vi "can test.vi"() -> ()   [LabVIEW 2015]
uses:
  <vilib>/FPGAPlugInAG/cRIO-9030/niLvFpga_Open_cRIO-9030.vi
  <vilib>/rvi/interface/common/dynamic/niFpgaDynamicAddResources.vi
  <vilib>/FPGAPlugInAG/Dynamic/niLvFpga_Abort_Dynamic.vi
  <vilib>/FPGAPlugInAG/Dynamic/niLvFpga_Run_Dynamic.vi
  <vilib>/Utility/error.llb/Error Cluster From Error Code.vi
  <vilib>/rvi/errors/niLvFpgaAdjustHostInterfaceError.vi
  <vilib>/rvi/interface/nirviOpenFPGA/nirviOpenFPGA.xnode
  FPGA Bitfiles/autonomous_FPGATarget4_fpga1_rudp+OsNkSQ.lvbitx
  samsung/fpga 1.vi
  <vilib>/rvi/interface/nirviMethod/nirviMethod.xnode
  <vilib>/FPGAPlugInAG/Dynamic/niLvFpga_ReadFifo_Dynamic.vi
  <vilib>/rvi/errors/niLvFpgaMergeErrorWithErrorCode.vi
  <vilib>/NI_Real-Time Target Support.lvlib
panel:
  out "tic":u32
  out "filesave":refnum<file>
  out "CAN_time 10":u32
  out "FPGA":refnum<k20>
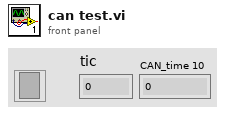
[diagram p1: front panel]
types:
  T1 = enum16{"open", "replace", "create", "open or create", "replace or create", "replace or create with confirmation"}
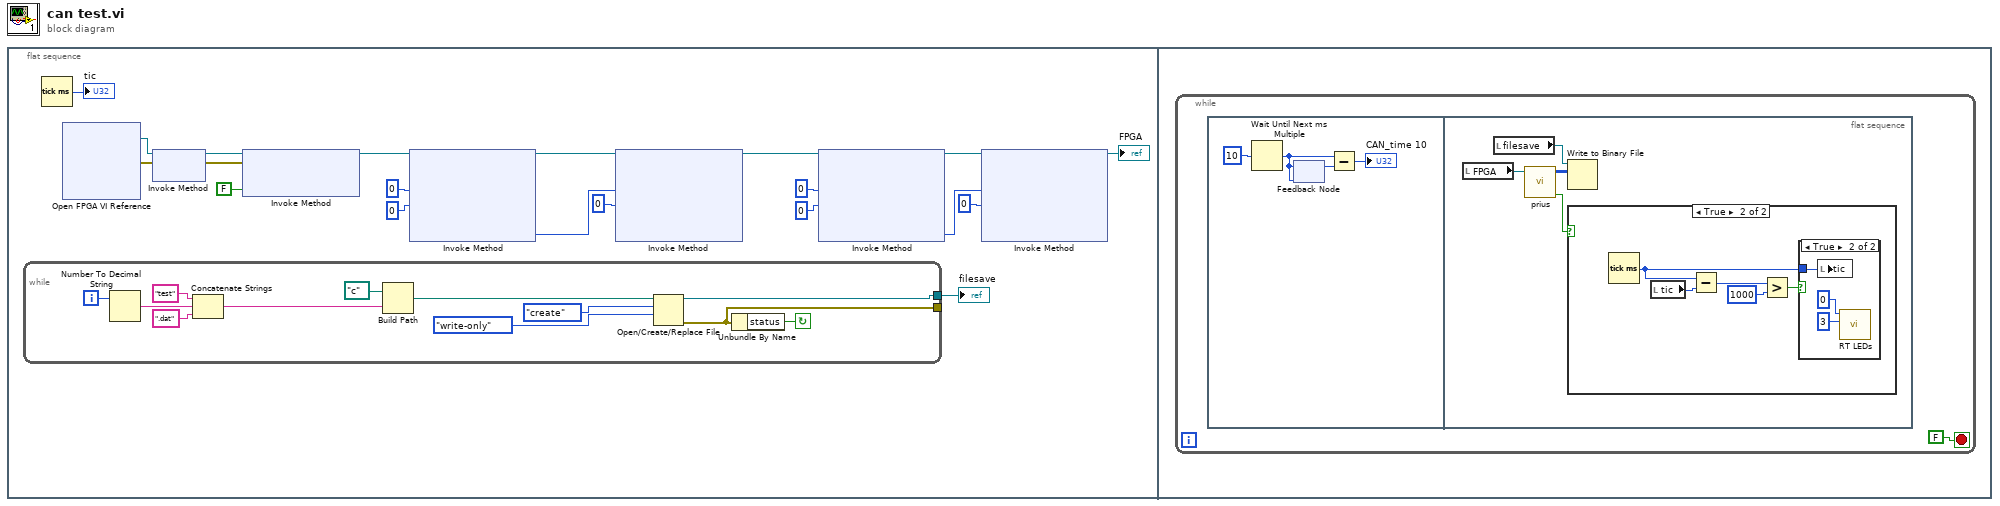
[diagram p0: block diagram]
diagram:
  n1 = flat-sequence {
    frame #0 {
      n2 = while {
        tunnel: [w31] -> w2
        tunnel: [w22] -> _
        i -> [w28]
        stop <- w21 continue-if-true
        n3 = Number To Decimal String(number=w28) -> (decimal integer string=w26:string)  [unwired: 1 in]
        n4 = Concatenate Strings("test" ("string"), w26, ".dat" ("string")) -> (w24:string)
        n5 = Build Path(base path=path "c:/" ("file path (use dialog)"), name or relative path=w24) -> (appended path=w27:path)
        n6 = Open/Create/Replace File(file path (use dialog)=w27, operation (0:open)=T1."create", access (0:read/write)=enum16{"read/write", "read-only", "write-only"}."write-only") -> (refnum out=w31:refnum<file>, error out=w22:errorcluster)  [unwired: 3 in, 1 out]
        n7 = Unbundle By Name(w22) -> ("status"=w21:bool)
      }
      "filesave" <- w2
      n8 = Tick Count (ms)() -> (millisecond timer value=→"tic":u32)
      n9 = xnode "Open FPGA VI Reference"() -> ("FPGA VI Reference Out"=w20:refnum<k20>, "error out"=w19:errorcluster)  [unwired: 2 in]
      n10 = xnode "Invoke Method"("FPGA VI Reference In"=w20, "error in"=w19) -> ("FPGA VI Reference Out"=w18:refnum<k20>, "error out"=w17:errorcluster)
      n11 = xnode "Invoke Method"("FPGA VI Reference In"=w18, "error in"=w17, "Wait Until Done (F)"=FALSE) -> ("FPGA VI Reference Out"=w15:refnum<k20>)  [unwired: 1 out]
      n12 = xnode "Invoke Method"("FPGA VI Reference In"=w15, "Number of Elements"=u32 0, "Timeout (ms)"=0) -> ("FPGA VI Reference Out"=w13:refnum<k20>, "Elements Remaining"=w12:u32)  [unwired: 1 in, 2 out]
      n13 = xnode "Invoke Method"("FPGA VI Reference In"=w13, "Number of Elements"=w12, "Timeout (ms)"=0) -> ("FPGA VI Reference Out"=w8:refnum<k20>)  [unwired: 1 in, 3 out]
      n14 = xnode "Invoke Method"("FPGA VI Reference In"=w8, "Number of Elements"=u32 0, "Timeout (ms)"=0) -> ("FPGA VI Reference Out"=w10:refnum<k20>, "Elements Remaining"=w11:u32)  [unwired: 1 in, 2 out]
      n15 = xnode "Invoke Method"("FPGA VI Reference In"=w10, "Number of Elements"=w11, "Timeout (ms)"=0) -> ("FPGA VI Reference Out"=→"FPGA":refnum<k20>)  [unwired: 1 in, 3 out]
    }
    frame #1 {
      n16 = while {
        stop <- FALSE stop-if-true
        n17 = flat-sequence {
          frame #0 {
            n18 = Wait Until Next ms Multiple(millisecond multiple=u32 10) -> (millisecond timer value=w35:u32)
            n19 = feedback #1(w35) -> (w36:u32)
            n20 = feedback-in #1(w35) -> ()
            n21 = Subtract(x=w35, y=w36) -> (x-y=→"CAN_time 10":u32)
          }
          frame #1 {
            n22 = local read "FPGA"() -> (w40:refnum<k20>)
            n23 = local read "filesave"() -> (w41:refnum<file>)
            n24 = call "prius.vi"("FPGA"=w40) -> ("can enabled"=w38:bool, "CAN Data"=w39:u8[][])  [unwired: 9 in]
            n25 = Write to Binary File(file (use dialog)=w41, data=w39) -> ()  [unwired: 4 in, 3 out]
            n26 = case shown="True" w38 {
              frame False {
              }
              frame True {
                n27 = Tick Count (ms)() -> (millisecond timer value=w45:u32)
                n28 = local read "tic"() -> (w42:u32)
                n29 = Subtract(x=w45, y=w42) -> (x-y=w43:u32)
                n30 = Greater?(x=w43, y=u32 1000) -> (0:w46:bool)
                n31 = case shown="True" w46 {
                  tunnel: w45 -> [_ w49]
                  frame False {
                  }
                  frame True {
                    n32 = local write "tic"(w49) -> ()
                    n33 = call <vilib>:"RT LEDs.vi"("State"=3, "LED Num"=0) -> ()  [unwired: 4 in, 2 out]
                  }
                }
              }
            }
          }
        }
      }
    }
  }
